vi "Log_Msg_Sub_VI.vi"(8 "Error In":errorcluster, 9 "Path for CSV":string="D:\\1. Darshan\\Ultrasonic_Test_Scripts\\Result_Next_Gen\\ResultTC_Get_last_weld_result_webserverDate_230719_Time_19_01_49.txt", 10 "String input":string, 11 "refnum in":refnum<file>) -> (0 "Error Out":errorcluster, 3 "refnum out":refnum<file>)   [LabVIEW 2017]
doc: "RESULT LOG:\nThis API is capable of storing results for all iterations after test case execution and able to create log.txt file at location as below\nand this log file will be uploded to RQM with execution record associated with the test case.\n \\Ultrasonic_Test_Scripts\\Result_Next_Gen\\ResultTC_TestcasenameDate_DDMMYY_Time_HH_MM_SS.txt\n\nFORMAT:\nIn below format results will be captured, user can always look at the results any time after test case execution\n\n[MM/SS/YYYY HH:MM:SS AM/PM] LabVIEW: #Datetime\nIteration# : N #Iterations\nWebserver response #Response from the webserver\nHeader: #Header for Debug purpose"
uses:
  <vilib>/Utility/file.llb/Write Delimited Spreadsheet (string).vi
panel:
  # "INPUT"
  # "ERROR"
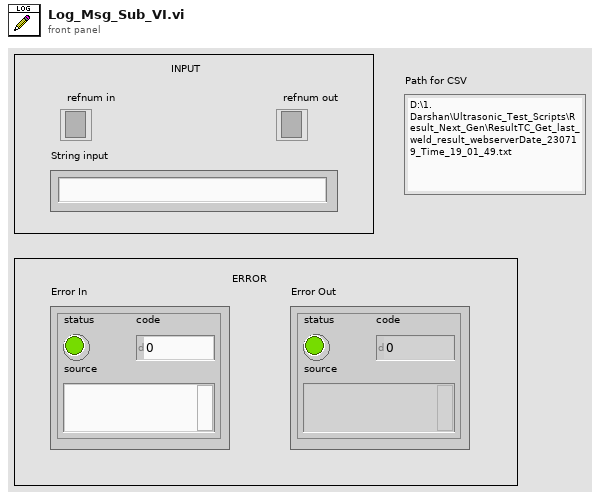
[diagram p1: front panel]
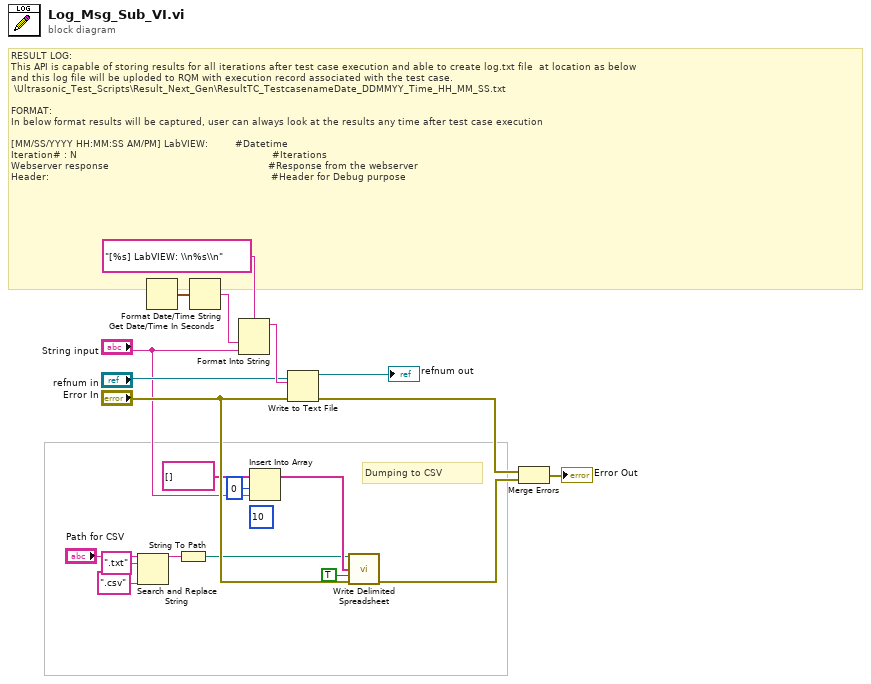
[diagram p0: block diagram]
diagram:
  (unwired) 10
  # "Dumping to CSV"
  # "RESULT LOG:\nThis API is capable of storing results for all iterations after test case execution and able to create log.txt file  at location as below\nand this log file will be uploded to RQM with execution record associated with the test case.\n \\Ultrasonic_Test_Scripts\\Result_Next_Gen\\ResultTC_TestcasenameDate_DDMMYY_Time_HH_MM_SS.txt\n\nFORMAT:\nIn below format results will be captured, user can always look at the results any time after test case execution\n\n[MM/SS/YYYY HH:MM:SS AM/PM] LabVIEW:         #Datetime\nIteration# : N                                                                 #Iterations\nWebserver response                                                     #Response from the webserver\nHeader:                                                                          #Header for Debug purpose"
  n1 = Search and Replace String(input string="Path for CSV", search string=".txt", replace string=".csv" ("replace string (\"\")")) -> (result string=w4:string)  [unwired: 5 in, 3 out]
  n2 = Get Date/Time In Seconds() -> (seconds since 1Jan1904=w17:timestamp)
  n3 = String To Path(string=w4) -> (path=w3:path)
  n4 = Format Date/Time String(seconds (now)=w17) -> (date/time string=w19:string)  [unwired: 2 out]
  n5 = Format Into String(format string="[%s] LabVIEW: \\n%s\\n", w19, "String input") -> (resulting string=w20:string)  [unwired: 2 in, 1 out]
  n6 = Insert Into Array(array=string[] [], index=0, new element="String input") -> (w8:string[])
  n7 = Write to Text File(file (use dialog)="refnum in", text=w20, error in="Error In") -> (refnum out=→"refnum out":refnum<file>, error out=w13:errorcluster)  [unwired: 2 out]
  n8 = call-poly <vilib>:"Write Delimited Spreadsheet.vi"("file path (dialog if empty)"=w3, "1D data"=w8, "append to file? (new file:F)"=TRUE, "error in (no error)"="Error In") -> ("error out"=w12:errorcluster)  [unwired: 10 in, 1 out]
  n9 = Merge Errors(w13, w12) -> (→"Error Out":errorcluster)
